vi "Setres_name.vi"(8 "error in (no error)":errorcluster, 10 "Set_Val":string, 11 "OneOfTemplate in":refnum<class "Greeter_res_res_oneof.lvclass">) -> (0 "error out":errorcluster, 3 "OneOfTemplate out":refnum<class "Greeter_res_res_oneof.lvclass">)   [LabVIEW 2019, in "Generated_server.lvlib" / "Greeter_res_res_oneof.lvclass"]
uses:
  Greeter_res_res_oneof.lvclass
  Greeter_res_res_oneof.lvclass/Greeter_res_res_oneof.ctl
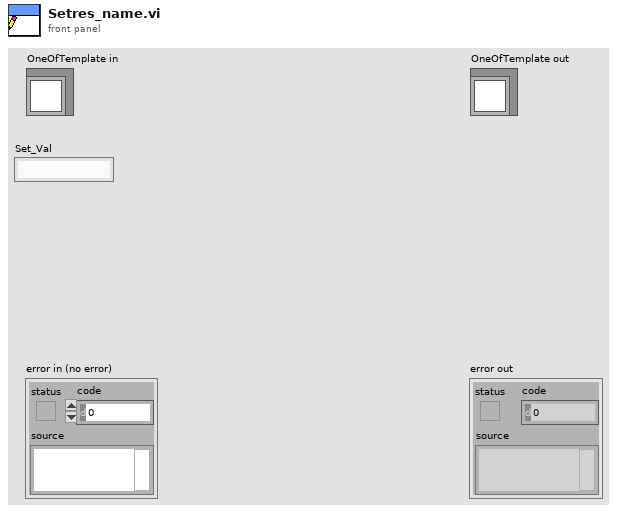
[diagram p1: front panel]
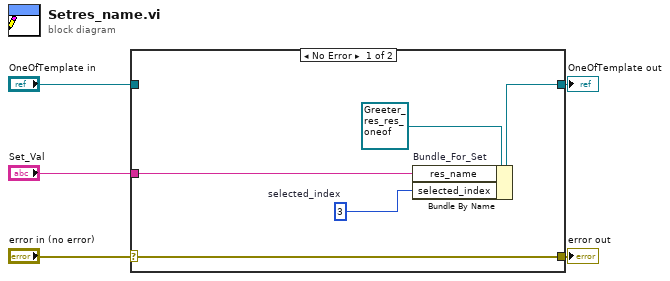
[diagram p0: block diagram]
diagram:
  n1 = case shown="No Error" "error in (no error)" {
    selector: "error in (no error)" -> [w10 w11]
    tunnel: [w10 w11] -> w4
    tunnel: [w9 w12] -> w2
    tunnel: "OneOfTemplate in" -> [_ w12]
    tunnel: "Set_Val" -> [w8 _]
    frame No Error {
      w7 = 3  # selected_index
      n2 = Bundle By Name "Bundle_For_Set"(cluster=refnum<class "Greeter_res_res_oneof.lvclass"> refnum ("OneOfTemplate in"), "res_name"=w8, "selected_index"=w7) -> (w9:refnum<class "Greeter_res_res_oneof.lvclass">)
    }
    frame Error {
    }
  }
  "error out" <- w4
  "OneOfTemplate out" <- w2
